vi "Destroy Session.vi"(8 "error in (no error)":errorcluster, 11 "net-http-client in":refnum<class "net-http-client.lvclass">) -> (0 "error out":errorcluster)   [LabVIEW 2020, in "net-http-client.lvclass"]
uses:
  net-http-client.lvclass
  net-http-client.lvclass/net-http-client.ctl
  <vilib>/Viviota/Viviota HTTP Client NET/LabVIEWHTTPClient_NET/HttpClient_NET.lvclass
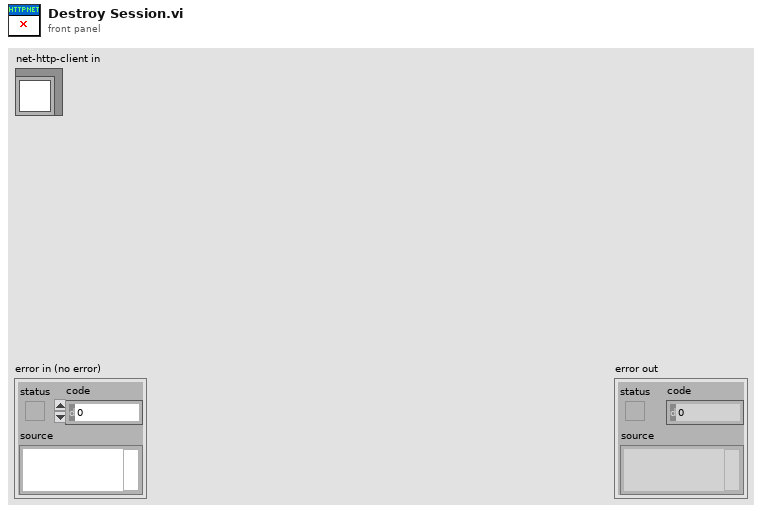
[diagram p1: front panel]
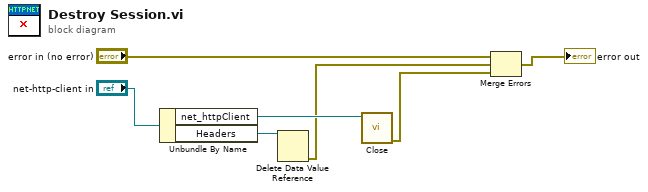
[diagram p0: block diagram]
diagram:
  n1 = Unbundle By Name("net-http-client in") -> ("net_httpClient"=w5:refnum<class "HttpClient_NET.lvclass">, "Headers"=w2:refnum<data-value>)
  n2 = Delete Data Value Reference(data value reference=w2) -> (error out=w1:errorcluster)  [unwired: 1 in, 1 out]
  n3 = call <vilib>:"Close.vi"("LabVIEWHTTPClient_NET in"=w5) -> ("Error Out"=w3:errorcluster)  [unwired: 10 in]
  n4 = Merge Errors("error in (no error)", w1, w3) -> (→"error out":errorcluster)
